vi "Move Turret.vi"(11 "CAN Talon SRX Ref":T1) -> (3 "Target X-value (norm)":dbl)   [LabVIEW 2016]
uses:
  <vilib>/Rock Robotics/WPI/MotorControl/WPI_MotorControlDeviceRef.ctl
  <vilib>/Rock Robotics/WPI/MotorControl/WPI_MotorControlType.ctl
  <vilib>/Rock Robotics/SystemInterfaces/DIO/FPGA_DIOPWMChannel.ctl
  <vilib>/Rock Robotics/WPI/PWM/WPI_PWMDeadband.ctl
  <vilib>/Rock Robotics/WPI/ThirdParty/CanMotor/TalonSRX/WPI_CANTalonSRX_APIControlMode.ctl
  Robot Global Data.vi
  <vilib>/Rock Robotics/Network Tables/NT Write Number.vi
panel:
  in  "Turret P":dbl=1.9 format="%#_13g"
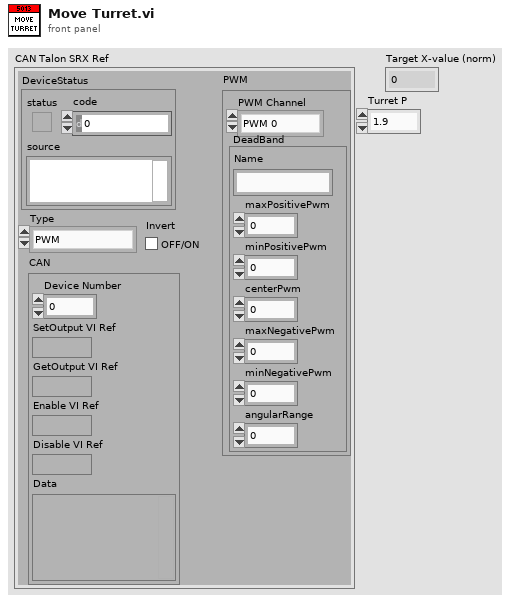
[diagram p1: front panel]
types:
  T1 = typedef "WPI_MotorControlDeviceRef.ctl" = cluster{"DeviceStatus":errorcluster, "Type":T2, "PWM":cluster{"PWM Channel":T3, "DeadBand":T4}, "CAN":cluster{"Device Number":u8, "SetOutput VI Ref":variant, "GetOutput VI Ref":variant, "Enable VI Ref":variant, "Disable VI Ref":variant, "Data":variant}, "Invert":bool}
  T2 = typedef "WPI_MotorControlType.ctl" = enum16{"PWM", "CAN"}
  T3 = typedef "FPGA_DIOPWMChannel.ctl" = enum8{"PWM 0", "PWM 1", "PWM 2", "PWM 3", "PWM 4", "PWM 5", "PWM 6", "PWM 7", "PWM 8", "PWM 9", "PWM MXP 0", "PWM MXP 1", "PWM MXP 2", "PWM MXP 3", "PWM MXP 4", "PWM MXP 5", "PWM MXP 6", "PWM MXP 7", "PWM MXP 8", "PWM MXP 9", "Invalid"}
  T4 = typedef "WPI_PWMDeadband.ctl" = cluster{"Name":string, "maxPositivePwm":i32, "minPositivePwm":i32, "centerPwm":i32, "maxNegativePwm":i32, "minNegativePwm":i32, "angularRange":u16}
  T5 = typedef "WPI_CANTalonSRX_APIControlMode.ctl" = enum8{"Percent VBus", "Speed", "Position", "Slave", "Unchanged / Invalid", "Voltage Compensation", "Current", "Motion Profile", "Motion Magic"}
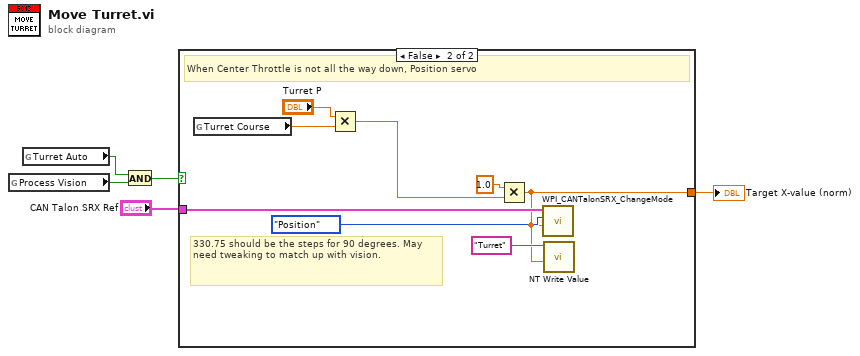
[diagram p0: block diagram]
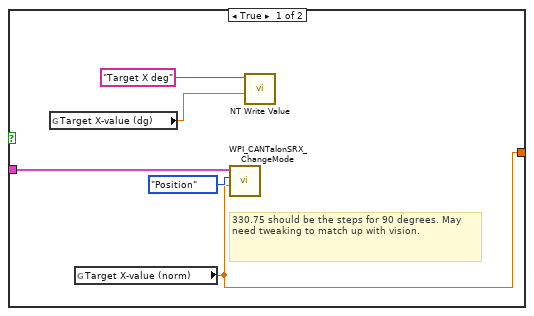
[diagram p2: hidden frame]
diagram:
  n1 = global read "Robot Global Data.vi" "Process Vision"() -> (w5:bool)
  n2 = global read "Robot Global Data.vi" "Turret Auto"() -> (w2:bool)
  n3 = And(x=w2, y=w5) -> (x .and. y?=w4:bool)
  n4 = case shown="False" w4 {
    tunnel: "CAN Talon SRX Ref" -> [w9 w17]
    tunnel: [w6 w11] -> w3
    frame True {
      # "330.75 should be the steps for 90 degrees. May need tweaking to match up with vision."
      n5 = global read "Robot Global Data.vi" "Target X-value (dg)"() -> (w7:dbl)
      n6 = global read "Robot Global Data.vi" "Target X-value (norm)"() -> (w6:dbl)
      n7 = call <vilib>:"WPI_CANTalonSRX_ChangeMode.vi"("Output"=w6, "Control Mode"=WPI_CANTalonSRX_APIControlMode."Position", "CAN Talon SRX Ref"=w9) -> ()  [unwired: 7 in, 2 out]
      n8 = call-poly <vilib>:"NT Write Value.vi"("Numeric"=w7, "Name"="Target X deg") -> ()  [unwired: 9 in, 1 out]
    }
    frame False {
      # "330.75 should be the steps for 90 degrees. May need tweaking to match up with vision."
      # "When Center Throttle is not all the way down, Position servo"
      n9 = global read "Robot Global Data.vi" "Turret Course"() -> (w15:dbl)
      n10 = Multiply(x="Turret P", y=w15) -> (x*y=w13:dbl)
      n11 = Multiply(x=1.0, y=w13) -> (x*y=w11:dbl)
      n12 = call <vilib>:"WPI_CANTalonSRX_ChangeMode.vi"("Output"=w11, "Control Mode"=WPI_CANTalonSRX_APIControlMode."Position", "CAN Talon SRX Ref"=w17) -> ()  [unwired: 7 in, 2 out]
      n13 = call-poly <vilib>:"NT Write Value.vi"("Numeric"=w11, "Name"="Turret") -> ()  [unwired: 9 in, 1 out]
    }
  }
  "Target X-value (norm)" <- w3
